vi "System Set Points and States.vi"() -> ()   [LabVIEW 2011]
uses:
  <vilib>/Rock Robotics/WPI/Joystick/WPI_JoystickButtonState.ctl
panel:
  out "LED blink rate":dbl
  out "Bridge Balance":bool
  in  "PID Stable":bool
  out "Auton":string
  out "CountDown":dbl
  out "Target Acquired":bool
  out "Locked On":bool
  out "Camera Enabled":bool
  out "Distance to Target":dbl
  out "Ball Count":dbl
  out "Loaded":bool
  out "Shooter Angle":dbl
  out "Axes":T1
  out "Buttons":T2
  out "Encoder Distance":dbl
  out "Left Encoder SetPoint":dbl
  out "Right Encoder SetPoint":dbl
  out "Indexer Dist":dbl
  out "Shooter RPM":dbl
  out "Indexer RPM":dbl
  out "Open Loop PWM":dbl
  in  "Open Loop":bool
  in  "Shooter Enabled":bool
  out "Hood Voltage":dbl
  out "ShooterSet Speed":dbl
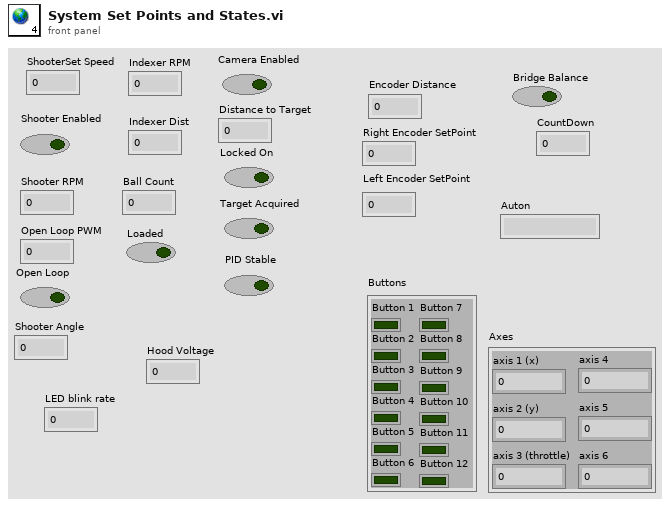
[diagram p1: front panel]
types:
  T1 = cluster{"axis 1 (x)":dbl, "axis 2 (y)":dbl, "axis 3 (throttle)":dbl, "axis 4":dbl, "axis 5":dbl, "axis 6":dbl}
  T2 = typedef "WPI_JoystickButtonState.ctl" = cluster{"Button 1":bool, "Button 2":bool, "Button 3":bool, "Button 4":bool, "Button 5":bool, "Button 6":bool, "Button 7":bool, "Button 8":bool, "Button 9":bool, "Button 10":bool, "Button 11":bool, "Button 12":bool}
diagram:
